vi "Write Control Limits.vi"(8 "error in":errorcluster, 10 "control limits":T1, 11 "Has Control Limits in":refnum<class "Has Control Limits.lvclass">) -> (0 "error out":errorcluster, 3 "Has Control Limits out":refnum<class "Has Control Limits.lvclass">)   [LabVIEW 2020, in "PV Access.lvlib" / "PV Data.lvlib" / "Has Control Limits.lvclass"]
uses:
  Has Control Limits.lvclass
  Control Metadata.ctl
  PV Data.lvlib
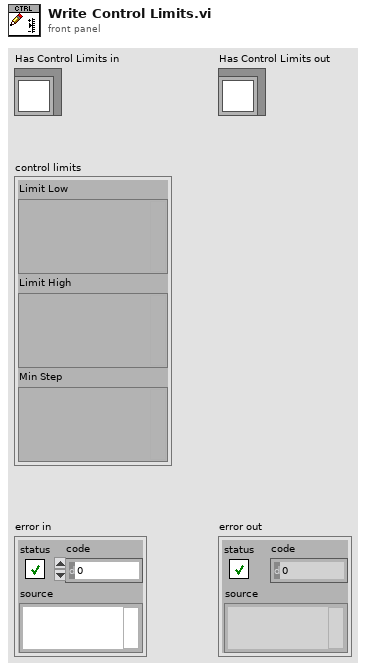
[diagram p1: front panel]
types:
  T1 = typedef "PV Access.lvlib/PV Data.lvlib/Control Metadata.ctl" = cluster{"Limit Low":variant, "Limit High":variant, "Min Step":variant}
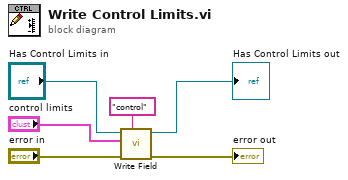
[diagram p0: block diagram]
diagram:
  n1 = call-dynamic "Write Field.vi"("field"="control", "error in (no error)"="error in", "value"="control limits", "Base Interface in"="Has Control Limits in") -> ("error out"=→"error out":errorcluster, "Base Interface out"=→"Has Control Limits out":refnum<class "Has Control Limits.lvclass">)  [unwired: 6 in]
